vi "Array2Excel.vi"(0 "text data":string[][](array[string]) caption="文本数据") -> ()   [LabVIEW 2015]
uses:
  <vilib>/Utility/NIReport.llb/Append Text Table to Report (wrap).vi
  <vilib>/Utility/NIReport.llb/NI_report.lvclass
  <vilib>/Utility/NIReport.llb/Excel/NI_Excel.lvclass
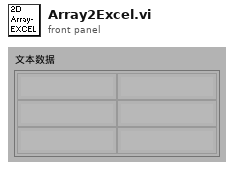
[diagram p1: front panel]
types:
  T1 = enum16{"Standard Report", "HTML", "Word", "Excel"}
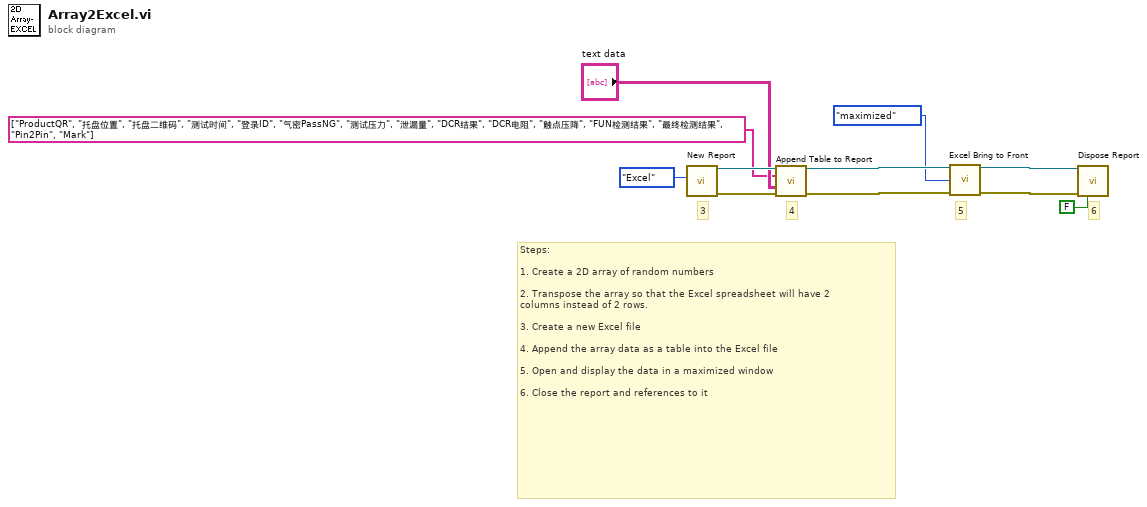
[diagram p0: block diagram]
diagram:
  # "6"
  # "5"
  # "4"
  # "3"
  # "Steps:\n\n1. Create a 2D array of random numbers\n\n2. Transpose the array so that the Excel spreadsheet will have 2 \ncolumns instead of 2 rows.\n\n3. Create a new Excel file\n\n4. Append the array data as a table into the Excel file\n\n5. Open and display the data in a maximized window\n\n6. Close the report and references to it"
  n1 = call <vilib>:"New Report.vi"("report type"=T1."Excel") -> ("report out"=w10:refnum<class "NI_report.lvclass">, "error out"=w9:errorcluster)  [unwired: 5 in, 8 out]
  n2 = call-poly <vilib>:"Append Table to Report.vi"("report in"=w10, "column headers"=string[] ["ProductQR", "托盘位置", "托盘二维码", "测试时间", "登录ID", "气密PassNG", "测试压力", "泄漏量", "DCR结果", "DCR电阻", "触点压降", "FUN检测结果", "最终检测结果", "Pin2Pin", "Mark"], "text data"="text data", "error in (no error)"=w9) -> ("report out"=w7:refnum<class "NI_report.lvclass">, "error out"=w6:errorcluster)  [unwired: 8 in, 2 out]
  n3 = call <vilib>:"Excel Bring to Front.vi"("report in"=w7, "window state (maximized)"=enum16{"maximized", "minimized", "normal"}."maximized", "error in (no error)"=w6) -> ("report out"=w4:refnum<class "NI_report.lvclass">, "error out"=w5:errorcluster)  [unwired: 11 out]
  n4 = call-dynamic "Dispose Report.vi"("report in"=w4, "error in (no error)"=w5, "close report? (T)"=FALSE) -> ()  [unwired: 2 in, 11 out]
